vi "Write DAQmx Config.vi"(8 "error in (no error)":errorcluster, 10 "DAQmxChannel":T1, 11 "configuration file path":path) -> (0 "error out":errorcluster)   [LabVIEW 2018]
doc: "Zapisuje do pliku ustawienia akwizycji dla karty DAQ"
uses:
  controls/daqtypedef.ctl
  <vilib>/Utility/config.llb/NI_LVConfig.lvlib
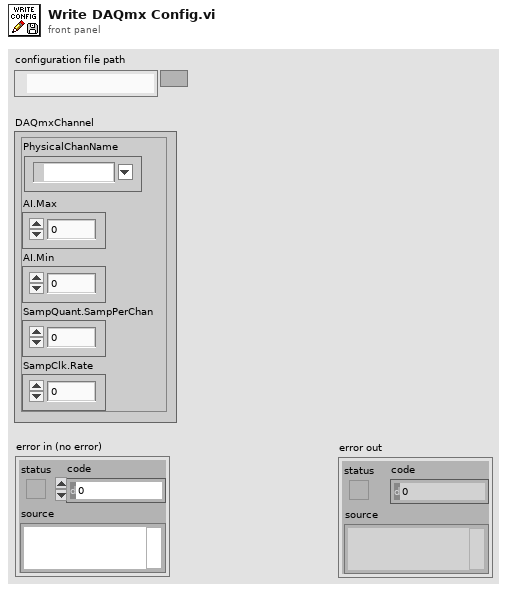
[diagram p1: front panel]
types:
  T1 = typedef "daqtypedef.ctl" = cluster{"PhysicalChanName":tag, "AI.Max":dbl, "AI.Min":dbl, "SampQuant.SampPerChan":dbl, "SampClk.Rate":dbl}
  T2 = typedef "NI_LVConfig.lvlib/Config Data RefNum.ctl" = refnum<k1>
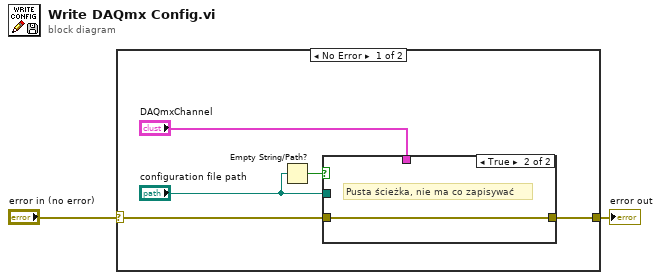
[diagram p0: block diagram]
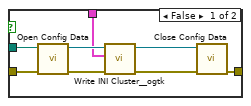
[diagram p2: hidden frame]
diagram:
  n1 = case shown="No Error" "error in (no error)" {
    selector: "error in (no error)" -> [w5 w17]
    tunnel: [w7 w17] -> w2
    frame No Error {
      n2 = Empty String/Path?(string/path="configuration file path") -> (empty?=w4:bool)
      n3 = case shown="True" w4 {
        tunnel: "configuration file path" -> [w14 _]
        tunnel: [w10 w16] -> w7
        tunnel: "DAQmxChannel" -> [w9 _]
        tunnel: w5 -> [w8 w16]
        frame False {
          n4 = call <vilib>:"Open Config Data.vi"("error in (no error)"=w8, "configuration file path"=w14) -> ("error out"=w15:errorcluster, "refnum"=w13:T2)  [unwired: 7 in, 1 out]
          n5 = call <userlib>:"Write INI Cluster__ogtk.vi"("error in (no error)"=w15, "INI Fomatted Cluster"=w9, "refnum"=w13) -> ("error out"=w12:errorcluster, "dup refnum"=w11:T2)  [unwired: 7 in]
          n6 = call <vilib>:"Close Config Data.vi"("error in (no error)"=w12, "refnum"=w11) -> ("error out"=w10:errorcluster)  [unwired: 8 in, 1 out]
        }
        frame True {
          # "Pusta ścieżka, nie ma co zapisywać"
        }
      }
    }
    frame Error {
    }
  }
  "error out" <- w2
